vi "Cockpit Cmd Inc.vi"(7 "Tip out Posit":dbl[](array[numeric])=[0.0, 0.0, 0.0] caption="Position [mm]" format="%#.3f", 8 "deltaRoll":sgl, 11 "deltaXYZ":sgl[](array[numeric])) -> (0 "Roll Out":sgl, 1 "Z Out":sgl, 2 "Y Out":sgl, 3 "X Out":sgl)   [LabVIEW 2016]
uses:
  Subsystems/Global Variables.vi
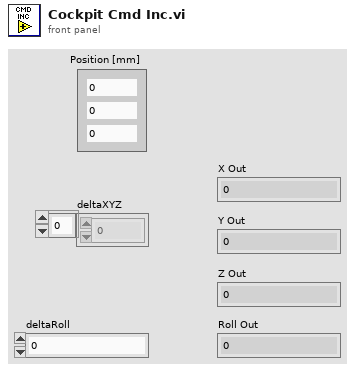
[diagram p1: front panel]
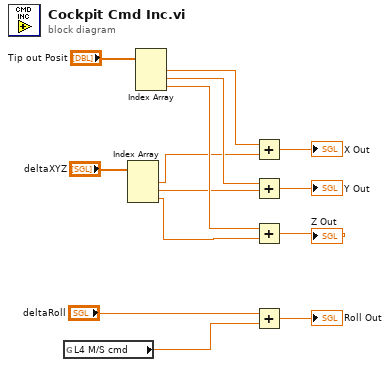
[diagram p0: block diagram]
diagram:
  n1 = global read "Global Variables.vi" "L4 M/S cmd"() -> (w13:dbl)
  n2 = Index Array(array="deltaXYZ") -> (element #1=w3:sgl, element #2=w2:sgl, element #3=w1:sgl)  [unwired: 3 in]
  n3 = Index Array(array="Tip out Posit") -> (element #1=w11:dbl, element #2=w9:dbl, element #3=w10:dbl)  [unwired: 3 in]
  n4 = Add(x=w11, y=w3) -> (x+y=→"X Out":dbl)
  n5 = Add(x=w9, y=w2) -> (x+y=→"Y Out":dbl)
  n6 = Add(x=w10, y=w1) -> (x+y=→"Z Out":dbl)
  n7 = Add(x="deltaRoll", y=w13) -> (x+y=→"Roll Out":dbl)
